vi "saveCSVCols.vi"(8 "Autosave":bool, 9 "y values":dbl[](array[numeric]), 10 "x":dbl, 11 "Image filename":path) -> ()   [LabVIEW 2012]
uses:
  <vilib>/Utility/file.llb/Write To Spreadsheet File (string).vi
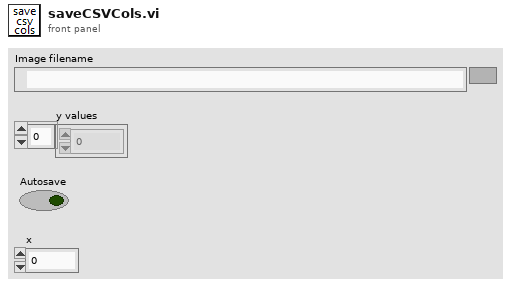
[diagram p1: front panel]
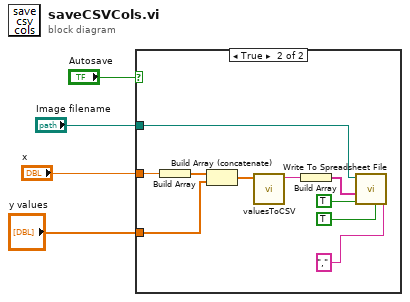
[diagram p0: block diagram]
diagram:
  n1 = case shown="True" "Autosave" {
    tunnel: "x" -> [_ w11]
    tunnel: "y values" -> [_ w9]
    tunnel: "Image filename" -> [_ w8]
    frame False {
    }
    frame True {
      n2 = Build Array(w11) -> (w10:dbl[])
      n3 = Build Array (concatenate)(w10, w9) -> (w7:dbl[])
      n4 = call "valuesToCSV.vi"("number"=w7) -> ("concatenated values"=w6:string)  [unwired: 10 in]
      n5 = Build Array(w6) -> (w5:string[])
      n6 = call-poly <vilib>:"Write To Spreadsheet File.vi"("delimiter (\\t)"="," ("delimiter (\\t)"), "transpose? (no:F)"=TRUE, "append to file? (new file:F)"=TRUE, "1D data"=w5, "file path (dialog if empty)"=w8) -> ()  [unwired: 3 in, 1 out]
    }
  }
